vi "CallUserScripting.vi"(8 "error in":errorcluster, 11 "ArrayElementScripter in":refnum<class "ArrayElementScripter.lvclass">) -> (0 "error out":errorcluster, 3 "ArrayElementScripter out":refnum<class "ArrayElementScripter.lvclass">)   [LabVIEW 2021, in "MemberVICreation.lvlib" / "ArrayElementScripter.lvclass"]
doc: "This VI provides an opportunity for users to add scripting code of their own to modify the scripting process even if they do not have the password to the VIs in the scripting. Each overriding class should call out to an empty subVI, one that is not a member of the class, that users can edit to put in their own scripting behavior."
uses:
  <resource>/Framework/Providers/LVClassLibrary/NewAccessors/ArrayElementScripter/ArrayElementScripter.lvclass
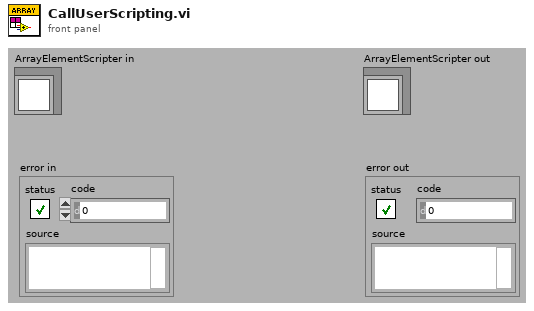
[diagram p1: front panel]
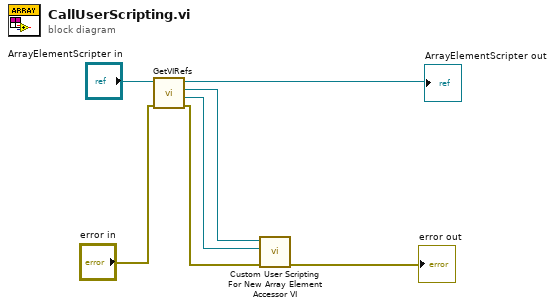
[diagram p0: block diagram]
diagram:
  n1 = call-dynamic "GetVIRefs.vi"("error in (no error)"="error in", "BaseAccessorScripter in"="ArrayElementScripter in") -> ("error out"=w4:errorcluster, "Write VI"=w3:refnum<vi>, "Read VI"=w2:refnum<vi>, "BaseAccessorScripter out"=→"ArrayElementScripter out":refnum<class "ArrayElementScripter.lvclass">)  [unwired: 6 in]
  n2 = call <resource>:"Custom User Scripting For New Array Element Accessor VI.vi"("error in"=w4, "Write VI"=w3, "Read VI"=w2) -> ("error out"=→"error out":errorcluster)  [unwired: 8 in]
